vi "Q8381 Head_Off and set Data.vi"(2 "Input String":string, 3 "Separater":string=",") -> (0 "Data":dbl[](array[numeric]) format="%.5e", 1 "Header":string)   [LabVIEW 2017]
doc: "If there is only one header at the biginning of input string, exclude the header and set remaining data to array."
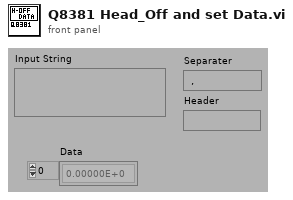
[diagram p1: front panel]
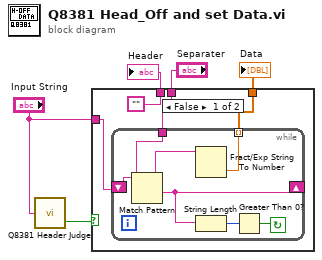
[diagram p0: block diagram]
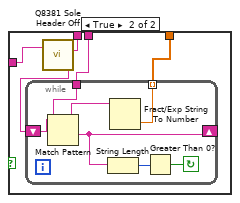
[diagram p2: hidden frame]
diagram:
  n1 = call "Q8381 Header Judge.vi"("String"="Input String") -> ("Output"=w1:bool)  [unwired: 1 out]
  n2 = case shown="False" w1 {
    tunnel: [w9 w21] -> w5
    tunnel: ["" w20] -> w3
    tunnel: "Separater" -> [w7 w18]
    tunnel: "Input String" -> [w6 w17]
    frame False {
      n3 = while {
        shift-right: [w15] -> _
        shift-left: w6 -> [w16]
        tunnel: [w11] -> w9 mode=indexing
        tunnel: w7 -> [w10]
        stop <- w13 continue-if-true
        n4 = Match Pattern(string=w16, regular expression=w10) -> (before substring=w12:string, after substring=w15:string)  [unwired: 1 in, 2 out]
        n5 = Fract/Exp String To Number(string=w12) -> (number=w11:dbl)  [unwired: 3 in, 1 out]
        n6 = String Length(string=w15) -> (length=w14:i32)
        n7 = Greater Than 0?(x=w14) -> (x > 0?=w13:bool)
      }
    }
    frame True {
      n8 = call "Q8381 Sole Header Off.vi"("Row Data"=w17) -> ("Header"=w20:string, "Head-Off Data"=w19:string)  [unwired: 2 in, 2 out]
      n9 = while {
        shift-right: [w27] -> _
        shift-left: w19 -> [w28]
        tunnel: [w23] -> w21 mode=indexing
        tunnel: w18 -> [w22]
        stop <- w25 continue-if-true
        n10 = Match Pattern(string=w28, regular expression=w22) -> (before substring=w24:string, after substring=w27:string)  [unwired: 1 in, 2 out]
        n11 = String Length(string=w27) -> (length=w26:i32)
        n12 = Fract/Exp String To Number(string=w24) -> (number=w23:dbl)  [unwired: 3 in, 1 out]
        n13 = Greater Than 0?(x=w26) -> (x > 0?=w25:bool)
      }
    }
  }
  "Data" <- w5
  "Header" <- w3
